vi "Storage index to Container.vi"(10 "Index":i32) -> (2 "Container":T1)   [LabVIEW 2015, in "cRIO-Carbondioxide.lvlib" / "CO2-Actor.lvlib" / "Storage Line.lvclass"]
uses:
  Storage Line.lvclass
  Controls/Sample Transfer Container Enumerator.ctl
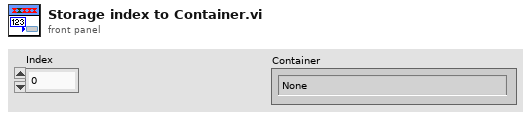
[diagram p1: front panel]
types:
  T1 = typedef "Sample Transfer Container Enumerator.ctl" = enum16{"None", "Sample 1", "Sample 2", "Sample 3", "Sample 4", "Sample 5", "Storage 01", "Storage 02", "Storage 03", "Storage 04", "Storage 05", "Storage 06", "Storage 07", "Storage 08", "Storage 09", "Storage 10", "Storage 11", "Storage 12", "Syringe", "Undefined"}
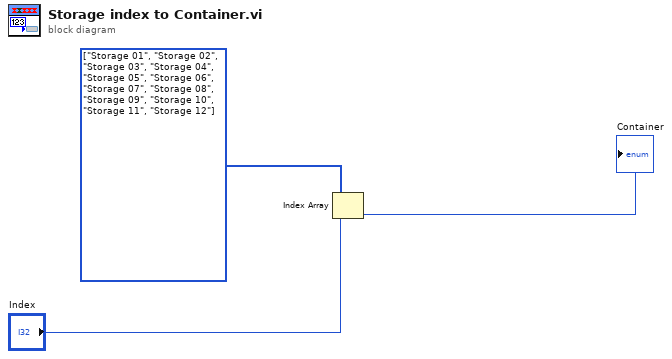
[diagram p0: block diagram]
diagram:
  w3 = T1[] [enum."Storage 01", enum."Storage 02", enum."Storage 03", enum."Storage 04", enum."Storage 05", enum."Storage 06", enum."Storage 07", enum."Storage 08", enum."Storage 09", enum."Storage 10", enum."Storage 11", enum."Storage 12"] items=["None", "Sample 1", "Sample 2", "Sample 3", "Sample 4", "Sample 5", "Storage 01", "Storage 02", "Storage 03", "Storage 04", "Storage 05", "Storage 06", "Storage 07", "Storage 08", "Storage 09", "Storage 10", "Storage 11", "Storage 12", "Syringe", "Undefined"]
  n1 = Index Array(array=w3, index="Index") -> (element=→"Container":T1)
